vi "Get Project Application Instance.vi"(8 "error in (no error)":errorcluster) -> (0 "error out":errorcluster, 3 "Application out":refnum<vi>)   [LabVIEW 2020]
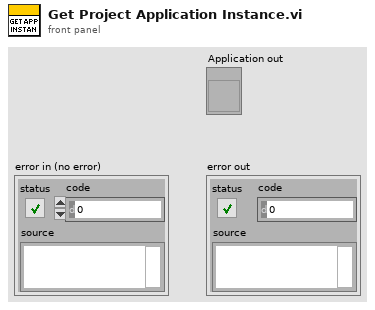
[diagram p1: front panel]
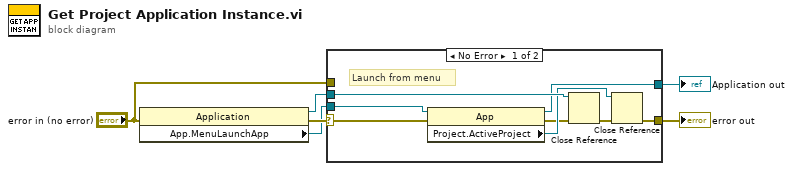
[diagram p0: block diagram]
diagram:
  n1 = property class="Application"(error in="error in (no error)") -> (reference out=w3:refnum<vi>, error out=w2:errorcluster, "App.MenuLaunchApp"=w1:refnum<vi>)  [unwired: 1 in]
  n2 = case shown="No Error" w2 {
    selector: w2 -> [w9 _]
    tunnel: [w12 w16] -> w5
    tunnel: w1 -> [w10 _]
    tunnel: [w7 w15] -> w6
    tunnel: "error in (no error)" -> [_ w15]
    tunnel: w3 -> [w14 w16]
    frame No Error {
      # "Launch from menu"
      n3 = property class="App"(reference=w10, error in=w9) -> (reference out=w12:refnum<vi>, error out=w11:errorcluster, "Project.ActiveProject"=w13:refnum<vi>)
      n4 = Close Reference(reference=w14, error in (no error)=w11) -> (error out=w8:errorcluster)
      n5 = Close Reference(reference=w13, error in (no error)=w8) -> (error out=w7:errorcluster)
    }
    frame Error {
    }
  }
  "error out" <- w6
  "Application out" <- w5
